vi "Continuous Setup.vi"(9 "measurement mode":T1 {"gain" max=15}, 10 "setup":T2={"integration time (s)"=0.5, "shortest wavelength"=190.0, "longest wavelength"=820.0, "sample interval (s)"=2.0, "delay (s)"=0.5} {"delay (s)" min=0 max=25.5 step=0.1 format="%.1f"; "sample interval (s)" min=1.1 max=99999.9 step=0.1 format="%.1f"; "longest wavelength" min=190 max=820 step=1; "shortest wavelength" min=190 max=820 step=1; "integration time (s)" min=0.1 max=25.5 step=0.1 format="%.1f"}, 11 "GPIB in":string="18") -> (0 "error occurred":bool, 3 "GPIB out":string="18")   [LabVIEW 2015]
uses:
  Continuous settings.ctl
  measurement mode.ctl
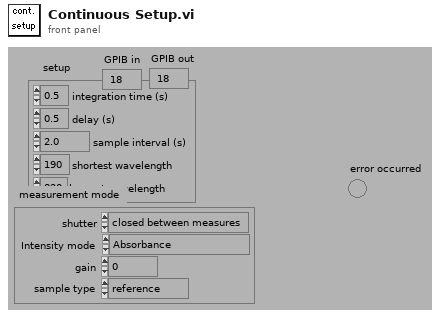
[diagram p1: front panel]
types:
  T1 = typedef "measurement mode.ctl" = cluster{"shutter":enum16{"closed between measures", "open between measures"}, "Intensity mode":enum16{"Absorbance", "Intensity at current gain", "Intensity at fixed gain", "dark current at current gain", "dark current at fixed gain"}, "gain":u8, "sample type":enum16{"reference", "standard", "unknown", "Diagnostic"}}
  T2 = typedef "Continuous settings.ctl" = cluster{"integration time (s)":sgl, "shortest wavelength":sgl, "longest wavelength":sgl, "sample interval (s)":dbl, "delay (s)":sgl}
  T3 = enum16{"closed between measures", "open between measures"}
  T4 = enum16{"Absorbance", "Intensity at current gain", "Intensity at fixed gain", "dark current at current gain", "dark current at fixed gain"}
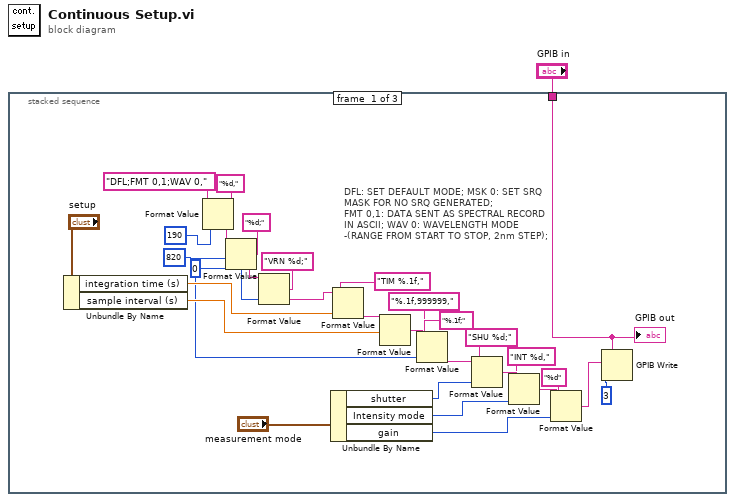
[diagram p0: block diagram]
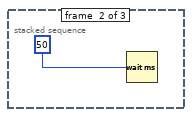
[diagram p2: hidden frame]
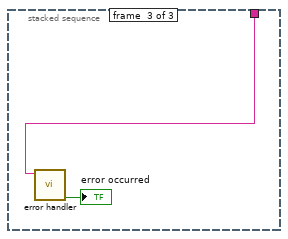
[diagram p3: hidden frame]
diagram:
  n1 = stacked-sequence {
    tunnel: "GPIB in" -> [w5 _ w34]
    frame #0 {
      w4 = 0
      # "DFL: SET DEFAULT MODE; MSK 0: SET SRQ\nMASK FOR NO SRQ GENERATED;\nFMT 0,1: DATA SENT AS SPECTRAL RECORD\nIN ASCII; WAV 0: WAVELENGTH MODE\n-(RANGE FROM START TO STOP, 2nm STEP);"
      n2 = Unbundle By Name("setup") -> ("integration time (s)"=w27:sgl, "sample interval (s)"=w28:dbl)
      n3 = Format Value(string ("")="DFL;FMT 0,1;WAV 0,", format string="%d,", value (0)=190) -> (output string=w8:string)
      n4 = Format Value(string ("")=w8, format string="%d;", value (0)=820) -> (output string=w10:string)
      n5 = Format Value(string ("")=w10, format string="VRN %d;", value (0)=w4) -> (output string=w12:string)
      n6 = Unbundle By Name("measurement mode") -> ("shutter"=w24:T3, "Intensity mode"=w25:T4, "gain"=w26:u8)
      n7 = Format Value(string ("")=w12, format string="TIM %.1f,", value (0)=w27) -> (output string=w14:string)
      n8 = Format Value(string ("")=w14, format string="%.1f,999999,", value (0)=w28) -> (output string=w30:string)
      n9 = Format Value(string ("")=w30, format string="%.1f;", value (0)=w4) -> (output string=w32:string)
      n10 = Format Value(string ("")=w32, format string="SHU %d;", value (0)=w24) -> (output string=w18:string)
      n11 = Format Value(string ("")=w18, format string="INT %d,", value (0)=w25) -> (output string=w19:string)
      n12 = Format Value(string ("")=w19, format string="%d", value (0)=w26) -> (output string=w21:string)
      n13 = GPIB Write(0:w5, 1:w21, 2:3) -> ()  [unwired: 2 in, 2 out]
      "GPIB out" <- w5
    }
    frame #1 {
      n14 = Wait (ms)(milliseconds to wait=50) -> ()  [unwired: 1 out]
    }
    frame #2 {
      n15 = call "error handler.vi"("GPIB in"=w34) -> ("error occurred"=→"error occurred":bool)  [unwired: 4 in, 2 out]
    }
  }
